vi "sendAllMessages.vi"(8 "error in (no error)":errorcluster, 11 "TCPServer in":refnum<class "TCPServer.lvclass">) -> (0 "error out":errorcluster, 3 "TCPServer out":refnum<class "TCPServer.lvclass">)   [LabVIEW 2016, in "TCPServer.lvclass"]
uses:
  TCPServer.lvclass
  C:/Users/aanania/Documents/ts_monochromator_windows/ts_labview_tcp/TCPCommunicator/TCPCommunicator.lvclass
  TCPCommunicator/TCPCommunicator.lvclass/TCPCommunicator.ctl
  TCPCommunicator/TCPCommunicator.lvclass
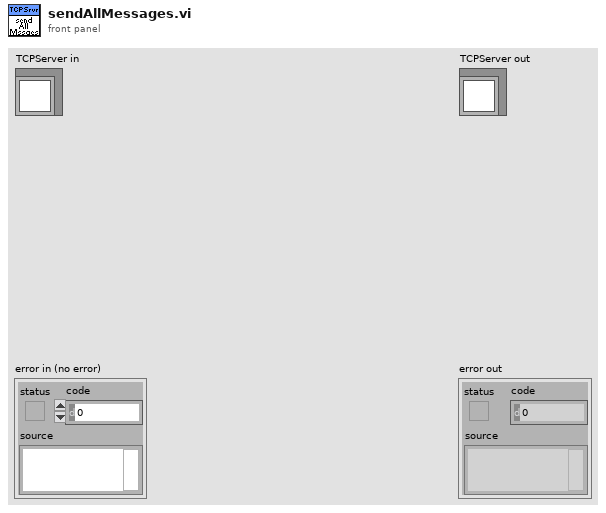
[diagram p1: front panel]
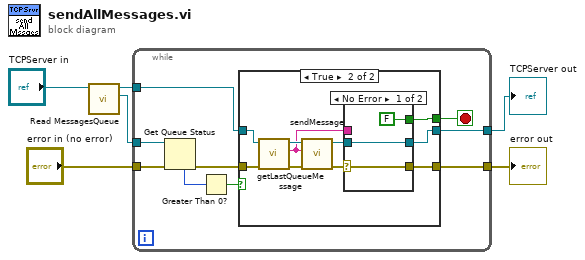
[diagram p0: block diagram]
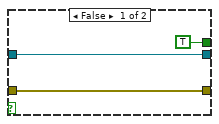
[diagram p2: hidden frame]
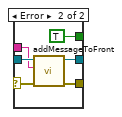
[diagram p3: hidden frame]
diagram:
  n1 = call "Read MessagesQueue.vi"("TCPCommunicator in"="TCPServer in") -> ("MessagesQueue"=w4:refnum<queue>, "TCPCommunicator out"=w3:refnum<class "TCPServer.lvclass">)  [unwired: 8 in, 1 out]
  n2 = while {
    tunnel: "error in (no error)" -> [w14]
    tunnel: [w13] -> w5
    tunnel: w4 -> [w9]
    tunnel: w3 -> [w8]
    tunnel: [w7] -> w1
    stop <- w10 stop-if-true
    n3 = Get Queue Status(queue=w9, error in (no error)=w14) -> (error out=w15:errorcluster, # elements in queue=w12:i32)  [unwired: 1 in, 6 out]
    n4 = Greater Than 0?(x=w12) -> (x > 0?=w11:bool)
    n5 = case shown="True" w11 {
      tunnel: w15 -> [w18 w28]
      tunnel: [w18 w23] -> w13
      tunnel: [TRUE w24] -> w10
      tunnel: w8 -> [w16 w26]
      tunnel: [w16 w19] -> w7
      frame False {
      }
      frame True {
        n6 = call "getLastQueueMessage.vi"("error in (no error)"=w28, "TCPCommunicator in"=w26) -> ("error out"=w27:errorcluster, "lastMessage"=w20:string, "TCPCommunicator out"=w25:refnum<class "TCPServer.lvclass">)  [unwired: 6 in, 1 out]
        n7 = call-dynamic "sendMessage.vi"("error in (no error)"=w27, "String"=w20, "TCPServer in"=w25) -> ("error out"=w22:errorcluster, "TCPServer out"=w21:refnum<class "TCPServer.lvclass">)  [unwired: 7 in]
        n8 = case shown="No Error" w22 {
          selector: w22 -> [w30 w34]
          tunnel: [FALSE TRUE] -> w24
          tunnel: [w30 w33] -> w23
          tunnel: w21 -> [w29 w36]
          tunnel: w20 -> [_ w35]
          tunnel: [w29 w32] -> w19
          frame No Error {
          }
          frame Error {
            n9 = call "addMessageToFront.vi"("error in (no error)"=w34, "message"=w35, "TCPCommunicator in"=w36) -> ("error out"=w33:errorcluster, "TCPCommunicator out"=w32:refnum<class "TCPServer.lvclass">)  [unwired: 6 in, 1 out]
          }
        }
      }
    }
  }
  "error out" <- w5
  "TCPServer out" <- w1
